vi "http read header.vi"(9 "default value":string, 10 "header field name":string, 11 "headers":T1) -> (1 "found":bool, 3 "value":string)   [LabVIEW 2016, in "http headers.lvlib"]
uses:
  http headers.lvlib
  http header data.ctl
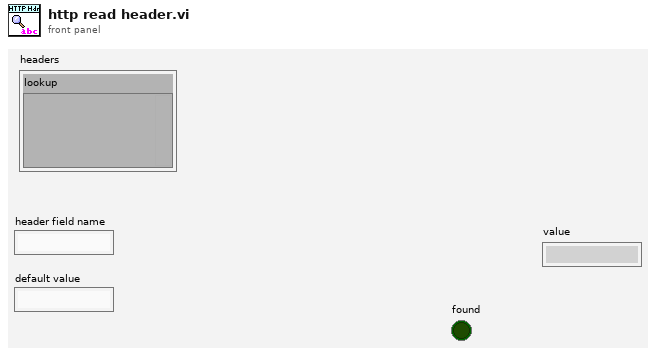
[diagram p1: front panel]
types:
  T1 = typedef "http headers.lvlib/http header data.ctl" = cluster{"lookup":variant}
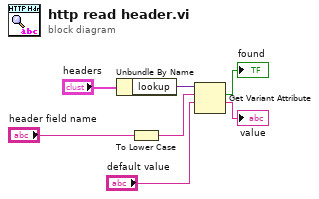
[diagram p0: block diagram]
diagram:
  n1 = Unbundle By Name("headers") -> ("lookup"=w5:variant)
  n2 = To Lower Case(string="header field name") -> (all lower case string=w4:string)
  n3 = Get Variant Attribute(Variant=w5, name=w4, default value (empty Variant)="default value") -> (found=→"found":bool, value=→"value":string)  [unwired: 1 in, 2 out]
